vi "Get XY.vi"(8 "error in (no error)":errorcluster, 10 "Channels":i32[](array[numeric])=[1], 11 "RP Instrument in":refnum<class "RP Instrument.lvclass">) -> (0 "error out":errorcluster, 1 "Y":i32=1 format="0x%x (%d)", 2 "X":i32=1 format="0x%x (%d)", 3 "RP Instrument out":refnum<class "RP Instrument.lvclass">)   [LabVIEW 2016, in "RP Instrument.lvclass"]
uses:
  RP Instrument.lvclass
  RP Status Offsets.ctl
  RP Instrument.lvclass/RP Instrument.ctl
  RP Communicator/RP Communicator.lvclass
panel:
  out "Array - Numeric":i32[](array[numeric]) format="0x%x (%d)"
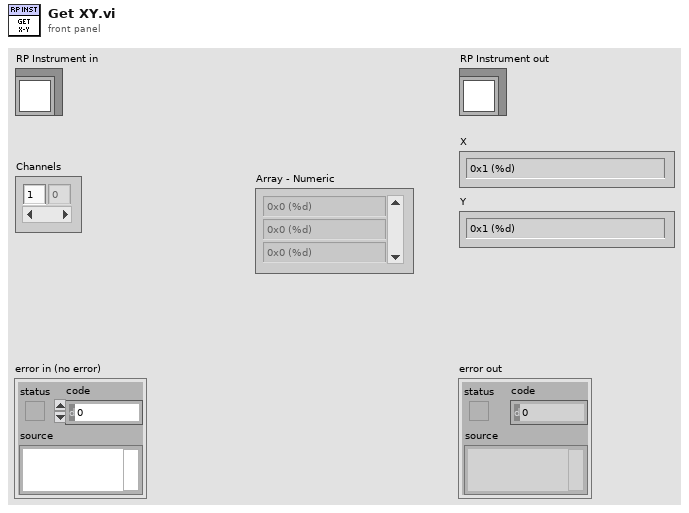
[diagram p1: front panel]
types:
  T1 = typedef "RP Status Offsets.ctl" = u16
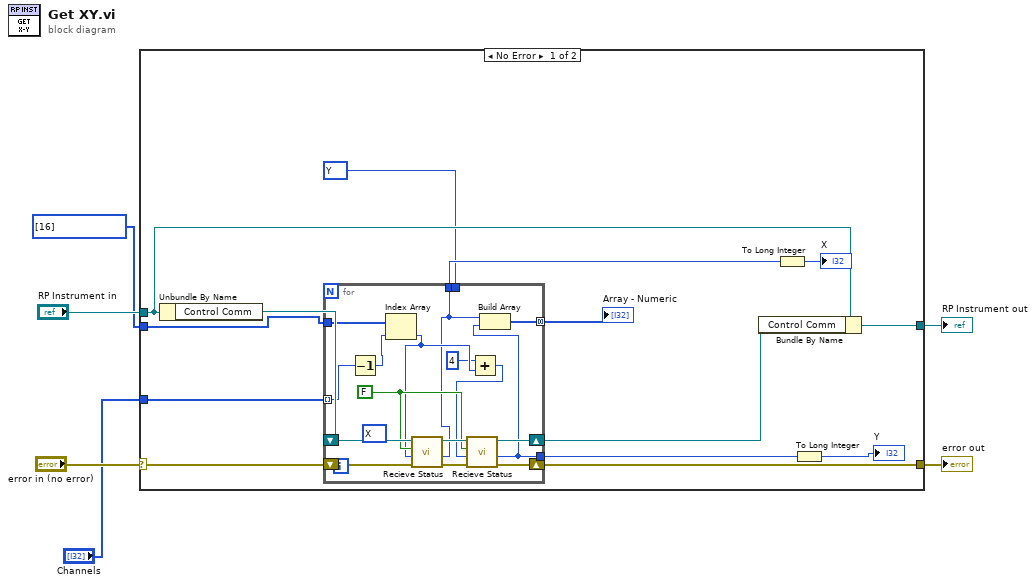
[diagram p0: block diagram]
diagram:
  n1 = case shown="No Error" "error in (no error)" {
    selector: "error in (no error)" -> [w19 w38]
    tunnel: [w15 w38] -> w5
    tunnel: [w16 w37] -> w3
    tunnel: "RP Instrument in" -> [w17 w37]
    tunnel: "Channels" -> [w9 _]
    tunnel: i64[] [16] -> [w8 _]
    frame No Error {
      w13 = T1 20 items=["Writer address"=0, "Record start position"=4, "Trig state and ID"=8, "Phase"=12, "X"=16, "Y"=20, "RxFIFO counter"=24, "TxFIFO counter"=28] ("Status offset")
      n2 = Unbundle By Name(w17) -> ("Control Comm"=w20:refnum<class "RP Communicator.lvclass">)
      n3 = for {
        tunnel: [w23] -> w18
        tunnel: w13 -> [_]
        tunnel: [w22] -> w12
        shift-right: [w31] -> w14
        shift-left: w20 -> [w36]
        shift-right: [w33] -> w15
        shift-left: w19 -> [w35]
        tunnel: w9 -> [w28] mode=indexing
        tunnel: w8 -> [w29]
        tunnel: [w21] -> w7 mode=concatenating
        (unwired) T1 16 items=["Writer address"=0, "Record start position"=4, "Trig state and ID"=8, "Phase"=12, "X"=16, "Y"=20, "RxFIFO counter"=24, "TxFIFO counter"=28] ("Status offset")
        w30 = FALSE ("Read config instead")
        n4 = Decrement(x=w28) -> (x-1=w27:i32)
        n5 = Index Array(array=w29, index=w27) -> (element=w26:i64)
        n6 = call-dynamic "Recieve Status.vi"("error in (no error)"=w35, "Status offset"=w26, "Read config instead"=w30, "RP Communicator in"=w36) -> ("error out"=w34:errorcluster, "Status response"=w23:u32, "RP Communicator out"=w32:refnum<class "RP Communicator.lvclass">)  [unwired: 5 in]
        n7 = Add(x=i64 4, y=w26) -> (x+y=w24:i64)
        n8 = call-dynamic "Recieve Status.vi"("error in (no error)"=w34, "Status offset"=w24, "Read config instead"=w30, "RP Communicator in"=w32) -> ("error out"=w33:errorcluster, "Status response"=w22:u32, "RP Communicator out"=w31:refnum<class "RP Communicator.lvclass">)  [unwired: 5 in]
        n9 = Build Array(w23, w22) -> (w21:u32[])
      }
      "Array - Numeric" <- w7
      n10 = Bundle By Name(cluster=w17, "Control Comm"=w14) -> (w16:refnum<class "RP Instrument.lvclass">)
      n11 = To Long Integer(number=w18) -> (32bit integer=→"X":i32)
      n12 = To Long Integer(number=w12) -> (32bit integer=→"Y":i32)
    }
    frame Error {
    }
  }
  "error out" <- w5
  "RP Instrument out" <- w3
